vi "getArrayValue.vi"(7 "Name":string, 8 "error in (no error)":errorcluster, 11 "tBSONDocument in":refnum<class "tBSONDocument.lvclass">) -> (0 "error out":errorcluster, 2 "Value":refnum<class "tBSONElement.lvclass">[](array[class]), 3 "tBSONDocument out":refnum<class "tBSONDocument.lvclass">)   [LabVIEW 2013, in "BSON.lvlib" / "tBSONDocument.lvclass"]
doc: "Retrieves an array of elements from a BSON document."
uses:
  tBSONDocument.lvclass
  tBSONElement/tBSONElement.lvclass
  BSONElements/tBSONArray/tBSONArray.lvclass
  BSONElements/tBSONArray/getValue.vi
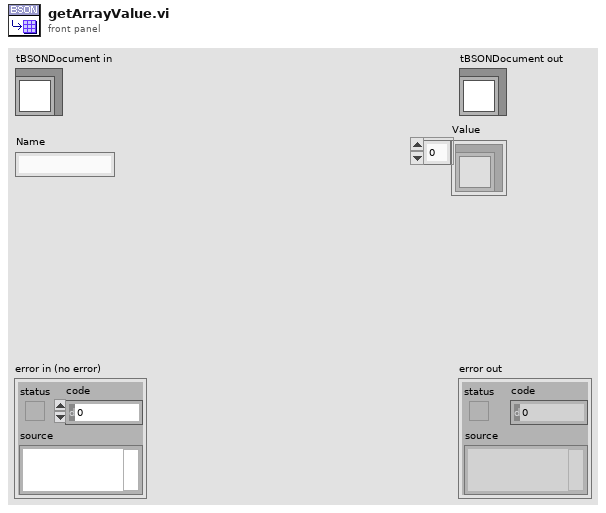
[diagram p1: front panel]
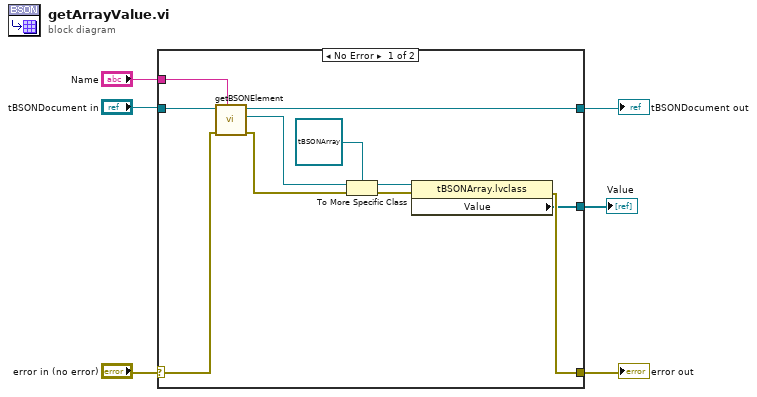
[diagram p0: block diagram]
diagram:
  n1 = case shown="No Error" "error in (no error)" {
    selector: "error in (no error)" -> [w16 w19]
    tunnel: [w10 w19] -> w2
    tunnel: [w11 w18] -> w3
    tunnel: "tBSONDocument in" -> [w17 w18]
    tunnel: "Name" -> [w7 _]
    tunnel: [w9 _] -> w1
    frame No Error {
      n2 = call "getBSONElement.vi"("Name"=w7, "error in (no error)"=w16, "tBSONDocument in"=w17) -> ("error out"=w12:errorcluster, "Element"=w13:refnum<class "tBSONElement.lvclass">, "tBSONDocument out"=w11:refnum<class "tBSONDocument.lvclass">)  [unwired: 6 in]
      n3 = To More Specific Class(target class=refnum<class "tBSONArray.lvclass"> refnum ("BSON.lvlib:tBSONArray.lvclass"), reference=w13, error in=w12) -> (specific class reference=w15:refnum<class "tBSONArray.lvclass">, error out=w14:errorcluster)
      n4 = property class="tBSONArray.lvclass"(reference=w15, error in=w14) -> (error out=w10:errorcluster, "Value"=w9:refnum<class "tBSONElement.lvclass">[])  [unwired: 1 out]
    }
    frame Error {
    }
  }
  "error out" <- w2
  "tBSONDocument out" <- w3
  "Value" <- w1
